vi "Create Connection.vi"(8 "error in (no error)":errorcluster, 11 "HostDB in":refnum<class "SQLite.lvclass">) -> (0 "error out":errorcluster, 3 "HostDB out":refnum<class "SQLite.lvclass">)   [LabVIEW 2017, in "SQLite.lvclass"]
uses:
  SQLite.lvclass
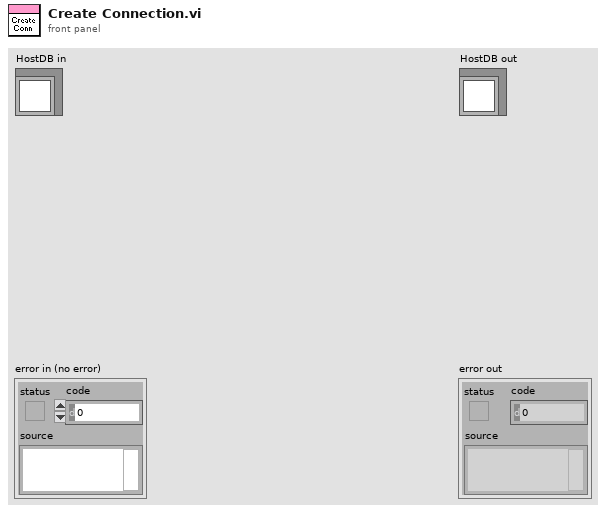
[diagram p1: front panel]
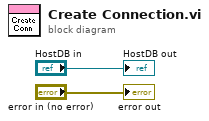
[diagram p0: block diagram]
diagram:
  "error out" <- "error in (no error)"
  "HostDB out" <- "HostDB in"
